vi "extuder main.vi"() -> ()   [LabVIEW 2014]
uses:
  <vilib>/Instr/_visa.llb/VISA Configure Serial Port (Instr).vi
panel:
  out "웨이브폼 차트 2":dbl(graph)
  out "숫자":dbl
  in  "Serial Port 2":refnum<visa-resource-name>="COM5"
  in  "압출기 (9600,8,E,1)":refnum<visa-resource-name>="COM4"
  in  "정지":bool
  out "해제":bool
  out "초기 위치":i32
  out "초기":bool
  out "Jog":bool
  out "설정":bool
  in  "클러스터":T1
  out "speed(r/min)":i32
  out "토크":i32(graph)
  in  "작동":bool
  out "토크 2":i32
  in  "정지 2":bool
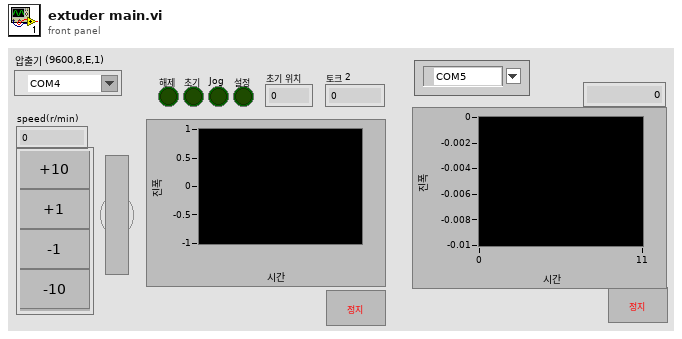
[diagram p1: front panel]
types:
  T1 = cluster{"+5":bool, "+1":bool, "-1":bool, "-5":bool}
  T2 = cluster{"국번":string, "커맨드":string, "데이터 No.":string, "데이터":string}
  T3 = cluster{"국번":string, "커맨드":string, "데이터 No.":string}
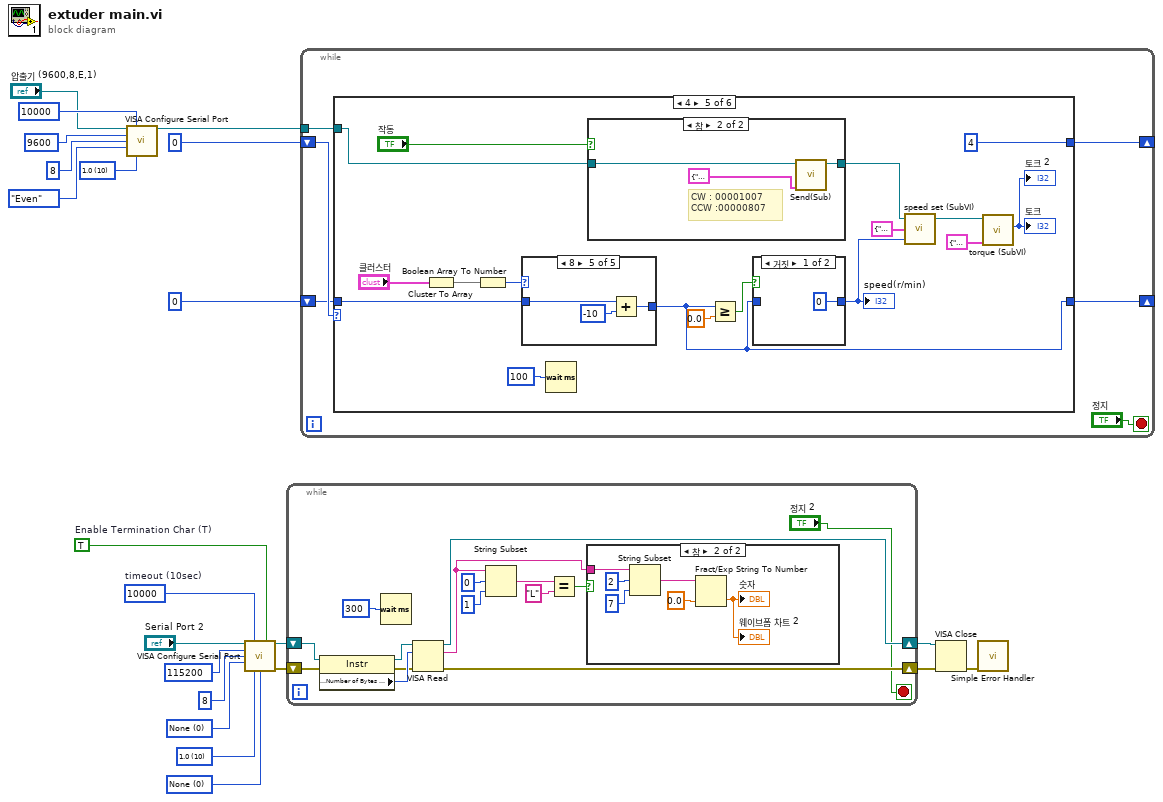
[diagram p0: block diagram]
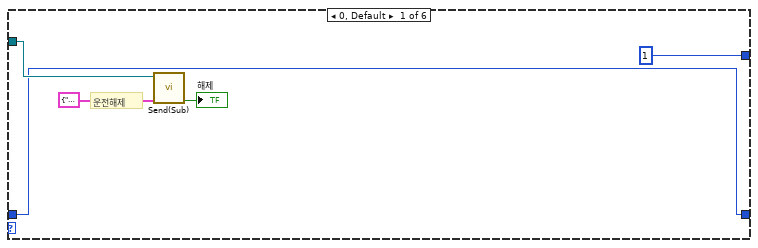
[diagram p2: hidden frame]
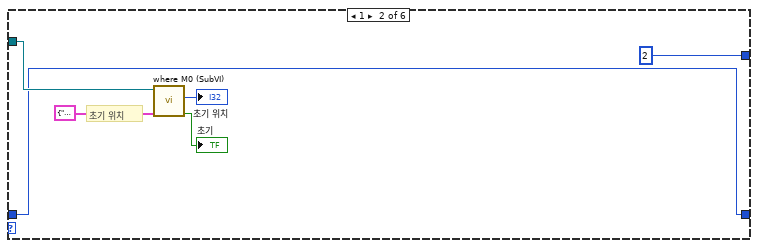
[diagram p3: hidden frame]
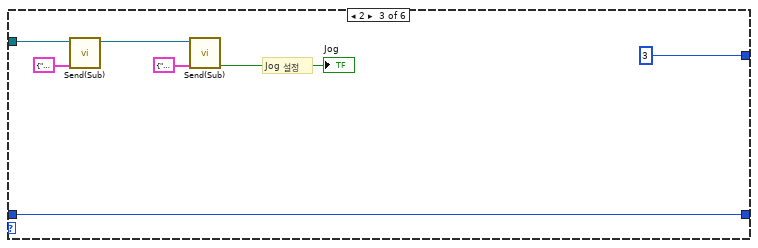
[diagram p4: hidden frame]
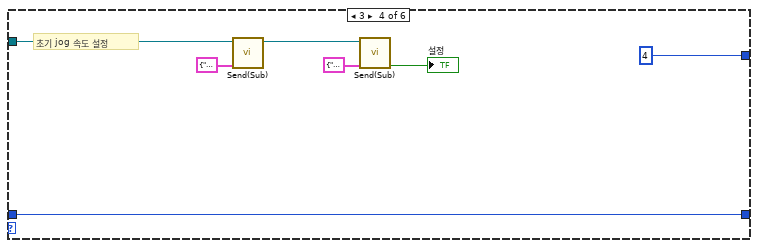
[diagram p5: hidden frame]
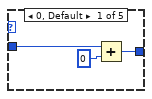
[diagram p7: hidden frame]
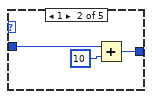
[diagram p8: hidden frame]
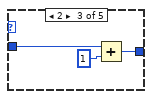
[diagram p9: hidden frame]
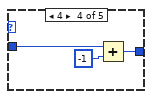
[diagram p10: hidden frame]
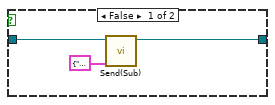
[diagram p11: hidden frame]
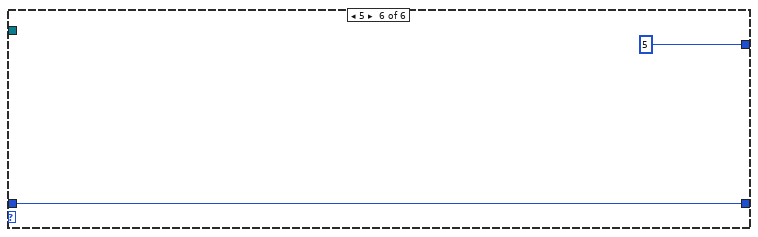
[diagram p12: hidden frame]
diagram:
  w8 = u16 10 items=["1.0"=10, "1.5"=15, "2.0"=20] ("stop bits (10: 1 bit)")
  w15 = u16 0 items=["None"=0, "XON/XOFF"=1, "RTS/CTS"=2, "DTR/DSR"=4] ("flow control")
  w16 = u16 10 items=["1.0"=10, "1.5"=15, "2.0"=20] ("stop bits")
  w19 = u16 0 items=["None", "Odd", "Even", "Mark", "Space"] ("parity")
  w17 = TRUE  # Enable Termination Char (T)
  w18 = u32 10000  # timeout (10sec)
  n1 = call-poly "VISA Configure Serial Port"("VISA resource name"="압출기 (9600,8,E,1)", "timeout (10sec)"=u32 10000, "baud rate (9600)"=u32 9600 ("baud rate"), "data bits (8)"=u16 8, "parity (0:none)"=enum16{"None", "Odd", "Even", "Mark", "Space"}."Even", "stop bits (10: 1 bit)"=w8) -> ("VISA resource name out"=w3:refnum<visa-resource-name>)  [unwired: 8 in, 1 out]
  n2 = call-poly "VISA Configure Serial Port"("VISA resource name"="Serial Port 2", "timeout (10sec)"=w18, "Enable Termination\nChar (T)"=w17, "baud rate (9600)"=u32 115200 ("baud rate"), "data bits (8)"=u16 8 ("data bits"), "parity (0:none)"=w19, "stop bits (10: 1 bit)"=w16, "flow control (0:none)"=w15) -> ("VISA resource name out"=w22:refnum<visa-resource-name>, "error out"=w21:errorcluster)  [unwired: 6 in]
  n3 = while {
    shift-right: [w34] -> w12
    shift-left: w22 -> [w31]
    shift-right: [w33] -> w11
    shift-left: w21 -> [w30]
    stop <- "정지 2" stop-if-true
    n4 = property class="Instr"(reference=w31, error in=w30) -> (reference out=w35:refnum<visa-resource-name>, error out=w36:errorcluster, "Serial Settings:Number of Bytes at Serial Port"=w37:u32)
    n5 = Wait (ms)(milliseconds to wait=u32 300 ("delay before\n read (ms)")) -> ()  [unwired: 1 out]
    n6 = VISA Read(VISA resource name=w35, byte count=w37, error in (no error)=w36) -> (VISA resource name out=w34:refnum<visa-resource-name>, read buffer=w24:string, error out=w33:errorcluster)  [unwired: 1 out]
    n7 = String Subset(string=w24, offset (0)=0 ("오프셋(0)"), length (rest)=1 ("길이(나머지)")) -> (substring=w25:string)
    n8 = Equal?(x=w25, y="L") -> (x = y?=w27:bool)
    n9 = case shown="참" w27 {
      tunnel: w24 -> [_ w40]
      frame False {
      }
      frame True {
        n10 = String Subset(string=w40, offset (0)=2 ("오프셋(0)"), length (rest)=7 ("길이(나머지)")) -> (substring=w41:string)
        n11 = Fract/Exp String To Number(string=w41, default (0 dbl)=0.0) -> (number=→"숫자" →"웨이브폼 차트 2":dbl)  [unwired: 2 in, 1 out]
      }
    }
  }
  n12 = while {
    tunnel: w3 -> [w49]
    shift-right: [w47] -> _
    shift-left: u16 0 ("data bits (8)") -> [w48]
    shift-right: [w44] -> _
    shift-left: u16 0 ("data bits (8)") -> [w45]
    stop <- "정지" stop-if-true
    n13 = case shown="4" w48 {
      tunnel: w49 -> [w53 w57 w63 w71 w86 _]
      tunnel: [u16 1 ("data bits (8)") u16 2 ("data bits (8)") u16 3 ("data bits (8)") u16 4 ("data bits (8)") u16 4 ("data bits (8)") u16 5 ("data bits (8)")] -> w47
      tunnel: w45 -> [w50 w55 w61 w68 w81 w115]
      tunnel: [w50 w55 w61 w68 w76 w115] -> w44
      frame 0, Default {
        # "운전해제"
        n14 = call "Send(Sub).vi"("보내기"=T2 {"국번"="0", "커맨드"="8B", "데이터 No."="00", "데이터"="0000"}, "VISA 참조 번호 입력"=w53) -> ("x = y?"=→"해제":bool)  [unwired: 7 in, 1 out]
      }
      frame 1 {
        # "초기 위치"
        n15 = call "where M0 (SubVI).vi"("요구"=T3 {"국번"="0", "커맨드"="01", "데이터 No."="80"}, "VISA 참조 번호 입력"=w57) -> ("x = y?"=→"초기":bool, "숫자 2"=→"초기 위치":i32)  [unwired: 4 in, 1 out]
      }
      frame 2 {
        # "Jog 설정"
        n16 = call "Send(Sub).vi"("보내기"=T2 {"국번"="0", "커맨드"="90", "데이터 No."="00", "데이터"="1EA5"}, "VISA 참조 번호 입력"=w63) -> ("VISA 참조 번호 출력"=w62:refnum<visa-resource-name>)  [unwired: 7 in, 1 out]
        n17 = call "Send(Sub).vi"("보내기"=T2 {"국번"="0", "커맨드"="8B", "데이터 No."="00", "데이터"="0001"}, "VISA 참조 번호 입력"=w62) -> ("x = y?"=→"Jog":bool)  [unwired: 7 in, 1 out]
      }
      frame 3 {
        # "초기 jog 속도 설정"
        n18 = call "Send(Sub).vi"("보내기"=T2 {"국번"="0", "커맨드"="A0", "데이터 No."="10", "데이터"="0000"}, "VISA 참조 번호 입력"=w71) -> ("VISA 참조 번호 출력"=w70:refnum<visa-resource-name>)  [unwired: 7 in, 1 out]
        n19 = call "Send(Sub).vi"("보내기"=T2 {"국번"="0", "커맨드"="A0", "데이터 No."="11", "데이터"="00000000"}, "VISA 참조 번호 입력"=w70) -> ("x = y?"=→"설정":bool)  [unwired: 7 in, 1 out]
      }
      frame 4 {
        n20 = Cluster To Array(cluster="클러스터") -> (array=w80:bool[])
        n21 = Boolean Array To Number(Boolean array=w80) -> (number=w78:u32)
        n22 = case shown="8" w78 {
          tunnel: [w95 w98 w102 w104 w107] -> w76
          tunnel: w81 -> [w94 w97 w100 w103 w106]
          frame 0, Default {
            n23 = Add(x=w94, y=0) -> (x+y=w95:i32)
          }
          frame 1 {
            n24 = Add(x=w97, y=10) -> (x+y=w98:i32)
          }
          frame 2 {
            n25 = Add(x=w100, y=1) -> (x+y=w102:i32)
          }
          frame 4 {
            n26 = Add(x=w103, y=-1) -> (x+y=w104:i32)
          }
          frame 8 {
            n27 = Add(x=w106, y=-10) -> (x+y=w107:i32)
          }
        }
        n28 = Wait (ms)(milliseconds to wait=u32 100 ("delay before read (ms)")) -> ()  [unwired: 1 out]
        n29 = case shown="참" "작동" {
          tunnel: w86 -> [w110 w113]
          tunnel: [w109 w112] -> w85
          frame False {
            n30 = call "Send(Sub).vi"("보내기"=T2 {"국번"="0", "커맨드"="92", "데이터 No."="00", "데이터"="00000007"}, "VISA 참조 번호 입력"=w110) -> ("VISA 참조 번호 출력"=w109:refnum<visa-resource-name>)  [unwired: 7 in, 1 out]
          }
          frame True {
            # "CW : 00001007\nCCW :00000807"
            n31 = call "Send(Sub).vi"("보내기"=T2 {"국번"="0", "커맨드"="92", "데이터 No."="00", "데이터"="00000807"}, "VISA 참조 번호 입력"=w113) -> ("VISA 참조 번호 출력"=w112:refnum<visa-resource-name>)  [unwired: 7 in, 1 out]
          }
        }
        n32 = Greater Or Equal?(x=w76, y=0.0) -> (x >= y?=w77:bool)
        n33 = case shown="거짓" w77 {
          tunnel: w76 -> [_ w93]
          tunnel: [0 w93] -> w75
          frame False {
          }
          frame True {
          }
        }
        "speed(r/min)" <- w75
        n34 = call "speed set (SubVI).vi"("speed(r/min)"=w75, "보내기"=T3 {"국번"="0", "커맨드"="A0", "데이터 No."="10"}, "VISA 참조 번호 입력"=w85) -> ("VISA 참조 번호 출력"=w88:refnum<visa-resource-name>)  [unwired: 1 in, 1 out]
        n35 = call "torque (SubVI).vi"("요구"=T3 {"국번"="0", "커맨드"="01", "데이터 No."="8A"}, "VISA 참조 번호 입력"=w88) -> ("숫자 2"=→"토크 2" →"토크":i32)  [unwired: 4 in, 2 out]
      }
      frame 5 {
      }
    }
  }
  n36 = VISA Close(VISA resource name=w12, error in (no error)=w11) -> (error out=w13:errorcluster)
  n37 = call <vilib>:"Simple Error Handler.vi"("error in (no error)"=w13) -> ()  [unwired: 4 in, 5 out]
